vi "Decreasing temp.vi"() -> ()   [LabVIEW 2016]
uses:
  <userlib>/Levylab/LV to ITX/LVtoITX.lvclass
  <vilib>/Analysis/NI_AALPro.lvlib
panel:
  out "appended array":dbl[][](array[numeric])
  out "M vs Temp Normalized 2":cluster{dbl[], dbl[]}[](graph)
  out "M vs Temp Normalized":cluster{dbl[], dbl[]}[](graph)
  out "output cluster":cluster{dbl[], dbl[], dbl[], dbl[]}
  in  "parameter bounds 2":T1={"slope min"=-inf, "slope max"=inf, "intercept min"=-inf, "intercept max"=inf}
  out "M vs Temp":T2(graph)
  out "Fits":T2(graph)
  out "Temp vs Time":cluster{"Data":dbl[], "Data":dbl[]}(graph)
  out "G vs Temp":cluster{"Data":dbl[], "Data":dbl[]}[](graph)
  in  "Path":path
  out "Wavenames":string[](array[string])
  out "Comments":string
  in  "header length":i32=11
  out "G vs Time":cluster{"Data":dbl[], "Data":dbl[]}[](graph)
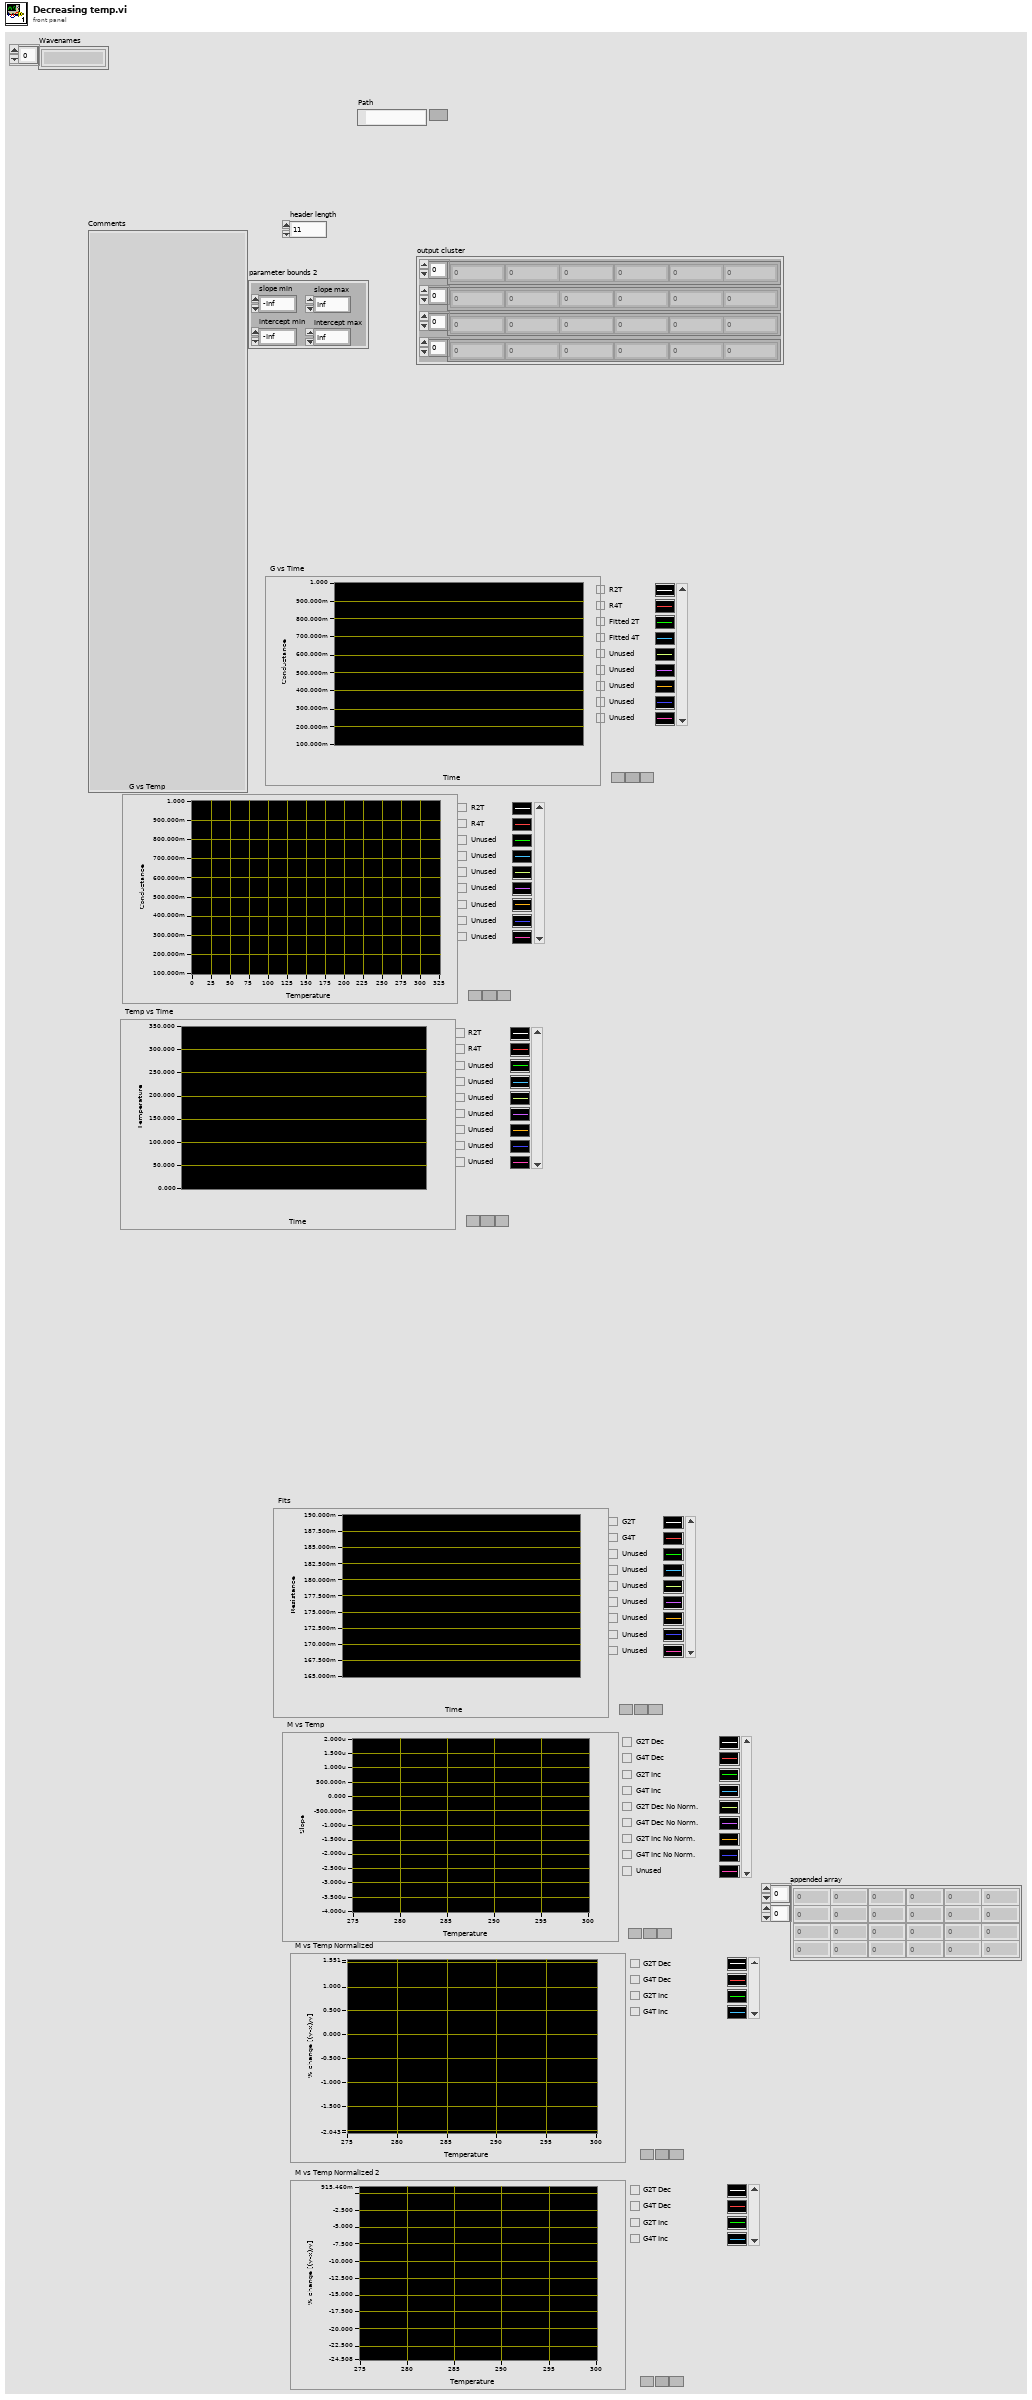
[diagram p1: front panel]
types:
  T1 = cluster{"slope min":dbl, "slope max":dbl, "intercept min":dbl, "intercept max":dbl}
  T2 = cluster{"Data":dbl[], "Best Exponential Fit":dbl[]}[]
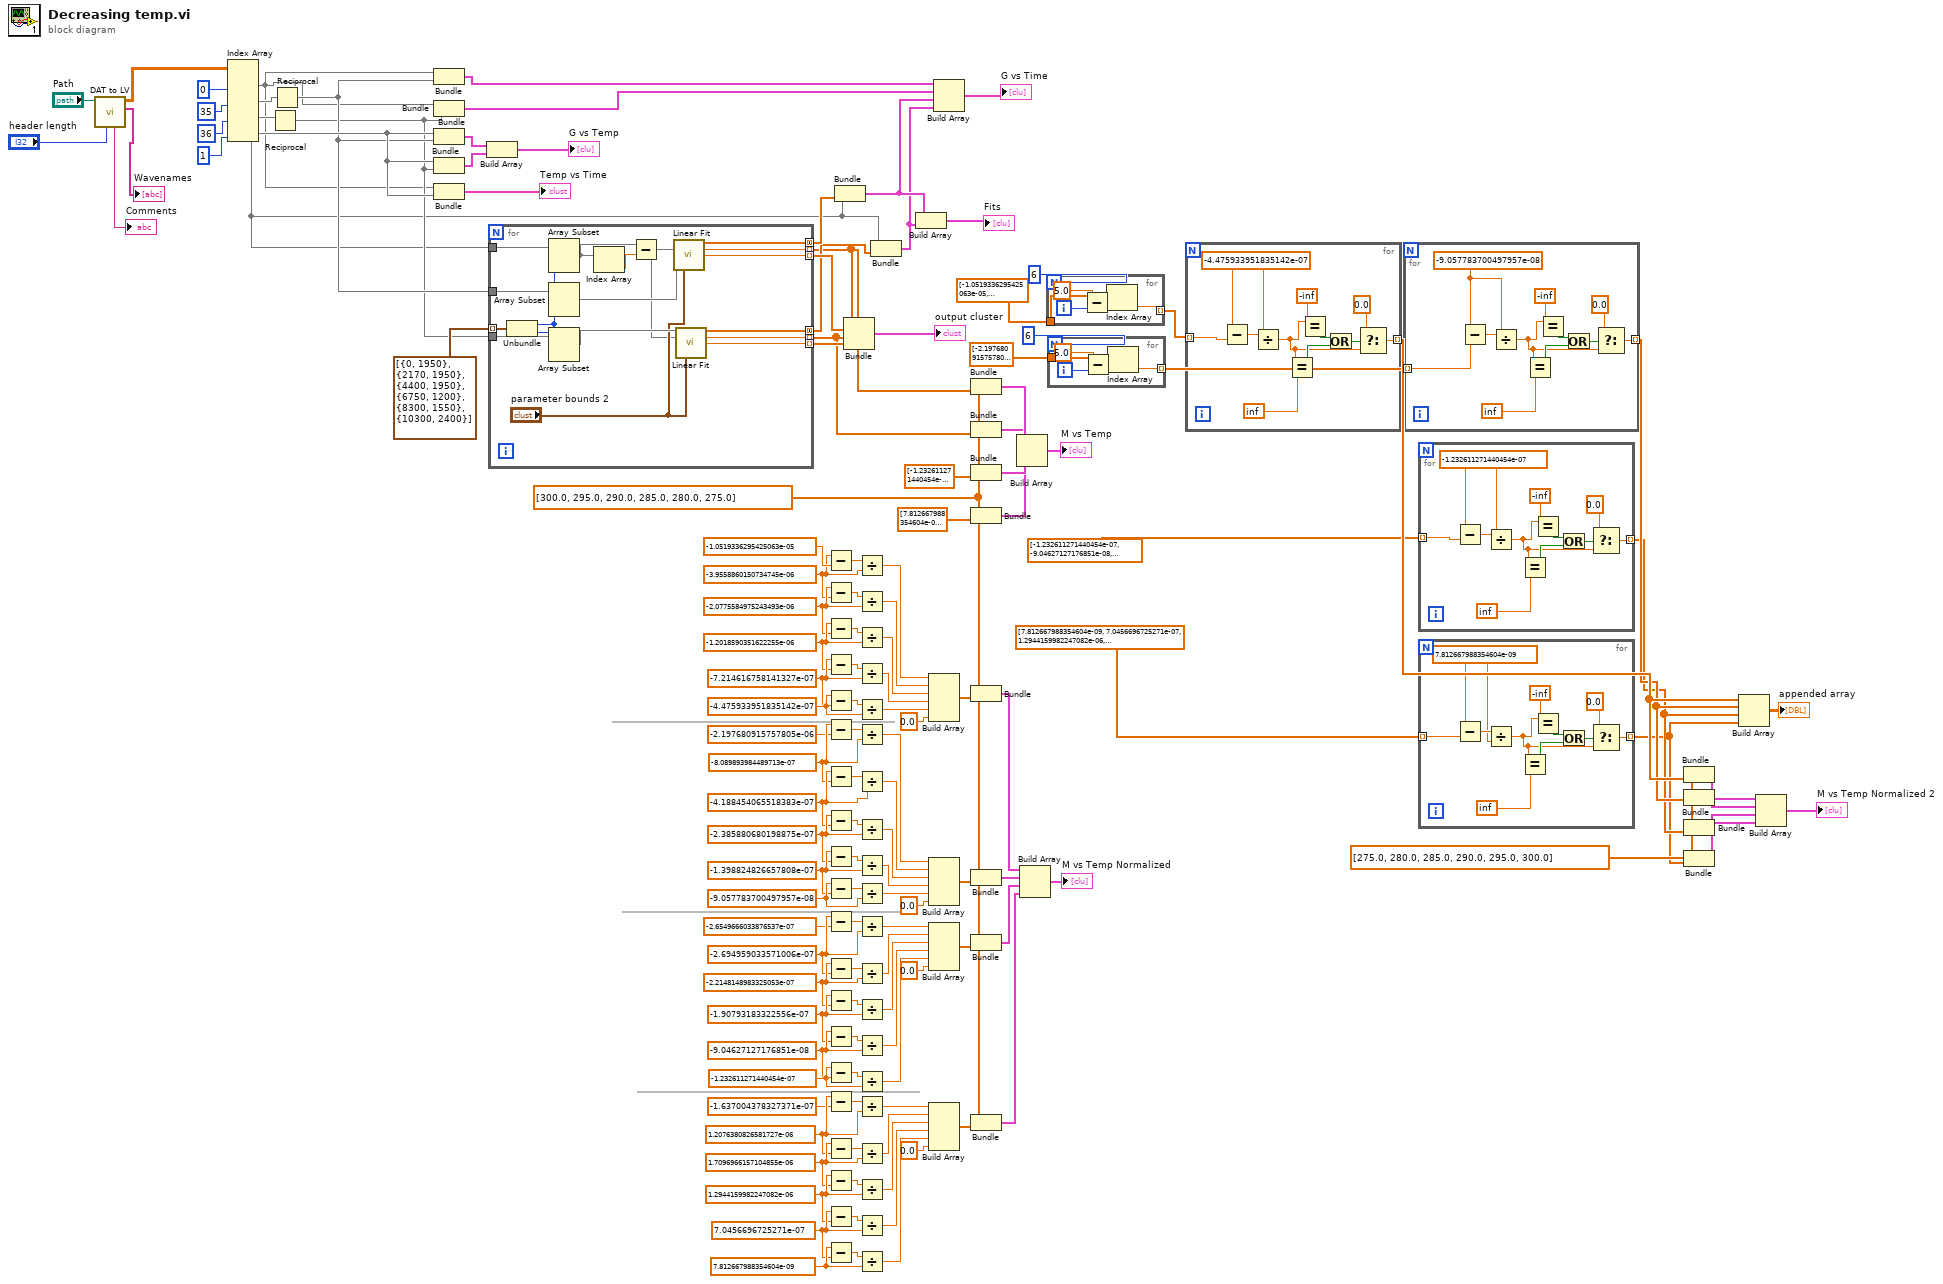
[diagram p0: block diagram]
diagram:
  w17 = dbl[] [275.0, 280.0, 285.0, 290.0, 295.0, 300.0]
  w29 = 1.2076380826581727e-06 ("slope")
  w30 = 1.7096966157104855e-06 ("slope")
  w31 = 1.2944159982247082e-06 ("slope")
  w32 = 7.0456696725271e-07 ("slope")
  w33 = 7.812667988354604e-09 ("slope")
  w46 = -2.694959033571006e-07 ("slope")
  w47 = -2.2148148983325053e-07 ("slope")
  w48 = -1.90793183322556e-07 ("slope")
  w49 = -9.04627127176851e-08 ("slope")
  w50 = -1.232611271440454e-07 ("slope")
  w67 = -9.057783700497957e-08 ("slope")
  w66 = -1.398824826657808e-07 ("slope")
  w65 = -2.385880680198875e-07 ("slope")
  w64 = -4.188454065518383e-07 ("slope")
  w63 = -8.089893984489713e-07 ("slope")
  w97 = -4.475933951835142e-07 ("slope")
  w95 = -7.214616758141327e-07 ("slope")
  w93 = -1.2018590351622255e-06 ("slope")
  w91 = -2.0775584975243493e-06 ("slope")
  w88 = -3.9558860150734745e-06 ("slope")
  w22 = dbl[] [300.0, 295.0, 290.0, 285.0, 280.0, 275.0]
  n1 = call <userlib>:"DAT to LV.vi"("header length"="header length", "File Path"="Path") -> ("Wavenames"=→"Wavenames":string[], "Data"=w129:dbl[][], "Comments"=→"Comments":string)  [unwired: 6 in, 1 out]
  n2 = Index Array(array=w129, index (col) #1=0 ("disabled index (col)"), index (col) #2=35 ("index (col)"), index (col) #3=36 ("index (col)"), index (col) #4=1 ("index (col)")) -> (element #1=w103:dbl[], element #2=w115:dbl[], element #3=w116:dbl[], element #4=w123:dbl[])  [unwired: 4 in]
  n3 = Reciprocal(x=w116) -> (1/x=w113:dbl[])
  n4 = Reciprocal(x=w115) -> (1/x=w114:dbl[])
  n5 = Bundle("Data"=w103, w114) -> (w128:cluster{"Data":dbl[], dbl[]})  [unwired: 1 in]
  n6 = Bundle("Data"=w103, w113) -> (w127:cluster{"Data":dbl[], dbl[]})  [unwired: 1 in]
  n7 = Bundle("Data"=w123, w114) -> (w125:cluster{"Data":dbl[], dbl[]})  [unwired: 1 in]
  n8 = Bundle("Data"=w123, w113) -> (w126:cluster{"Data":dbl[], dbl[]})  [unwired: 1 in]
  n9 = Bundle("Data"=w103, "Data"=w123) -> (→"Temp vs Time":cluster{"Data":dbl[], "Data":dbl[]})  [unwired: 1 in]
  n10 = Build Array(w125, w126) -> (→"G vs Temp":cluster{"Data":dbl[], dbl[]}[])
  n11 = for {
    tunnel: cluster{"index":i32, "length":i32}[] [{"index"=0, "length"=1950}, {"index"=2170, "length"=1950}, {"index"=4400, "length"=1950}, {"index"=6750, "length"=1200}, {"index"=8300, "length"=1550}, {"index"=10300, "length"=2400}] -> [w155] mode=indexing
    tunnel: [w154] -> w98 mode=indexing
    tunnel: [w153] -> w120 mode=indexing
    tunnel: [w152] -> w99 mode=indexing
    tunnel: [w151] -> w118 mode=indexing
    tunnel: [w150] -> w100 mode=concatenating
    tunnel: [w149] -> w121 mode=concatenating
    tunnel: w114 -> [w147]
    tunnel: w113 -> [w146]
    tunnel: w103 -> [w142]
    n12 = Unbundle(w155) -> ("index"=w141:i32, "length"=w148:i32)
    n13 = Array Subset(array=w142, index=w141, length=w148) -> (w139:dbl[])
    n14 = Array Subset(array=w147, index=w141, length=w148) -> (w144:dbl[])
    n15 = Array Subset(array=w146, index=w141, length=w148) -> (w145:dbl[])
    n16 = Index Array(array=w139) -> (element=w140:dbl)  [unwired: 1 in]
    n17 = Subtract(x=w139, y=w140) -> (x-y=w138:dbl[])
    n18 = call <vilib>:"Linear Fit.vi"("Y"=w144, "X"=w138, "parameter bounds"="parameter bounds 2") -> ("Best Linear Fit"=w149:dbl[], "slope"=w154:dbl, "intercept"=w153:dbl)  [unwired: 8 in, 2 out]
    n19 = call <vilib>:"Linear Fit.vi"("Y"=w145, "X"=w138, "parameter bounds"="parameter bounds 2") -> ("Best Linear Fit"=w150:dbl[], "slope"=w152:dbl, "intercept"=w151:dbl)  [unwired: 8 in, 2 out]
  }
  n20 = Subtract(x=w88, y=-1.0519336295425063e-05 ("slope")) -> (x-y=w87:dbl)
  n21 = Subtract(x=w91, y=w88) -> (x-y=w90:dbl)
  n22 = Subtract(x=w93, y=w91) -> (x-y=w92:dbl)
  n23 = Subtract(x=w95, y=w93) -> (x-y=w94:dbl)
  n24 = Subtract(x=w97, y=w95) -> (x-y=w96:dbl)
  n25 = Subtract(x=w63, y=-2.197680915757805e-06 ("slope")) -> (x-y=w72:dbl)
  n26 = Subtract(x=w64, y=w63) -> (x-y=w71:dbl)
  n27 = Subtract(x=w65, y=w64) -> (x-y=w70:dbl)
  n28 = Subtract(x=w66, y=w65) -> (x-y=w69:dbl)
  n29 = Subtract(x=w67, y=w66) -> (x-y=w68:dbl)
  n30 = Subtract(x=w46, y=-2.6549666033876537e-07 ("slope")) -> (x-y=w57:dbl)
  n31 = Subtract(x=w47, y=w46) -> (x-y=w58:dbl)
  n32 = Subtract(x=w48, y=w47) -> (x-y=w59:dbl)
  n33 = Subtract(x=w49, y=w48) -> (x-y=w60:dbl)
  n34 = Subtract(x=w50, y=w49) -> (x-y=w61:dbl)
  n35 = Subtract(x=w29, y=-1.637004378327371e-07 ("slope")) -> (x-y=w38:dbl)
  n36 = Subtract(x=w30, y=w29) -> (x-y=w37:dbl)
  n37 = Subtract(x=w31, y=w30) -> (x-y=w36:dbl)
  n38 = Subtract(x=w32, y=w31) -> (x-y=w35:dbl)
  n39 = Subtract(x=w33, y=w32) -> (x-y=w34:dbl)
  n40 = Bundle("Data"=w103, "Best Linear Fit"=w121) -> (w112:cluster{"Data":dbl[], "Best Linear Fit":dbl[]})  [unwired: 1 in]
  n41 = Bundle(w98, w120, w99, w118) -> (→"output cluster":cluster{dbl[], dbl[], dbl[], dbl[]})  [unwired: 1 in]
  n42 = Divide(x=w87, y=w88) -> (x/y=w85:dbl)
  n43 = Divide(x=w90, y=w91) -> (x/y=w84:dbl)
  n44 = Divide(x=w92, y=w93) -> (x/y=w83:dbl)
  n45 = Divide(x=w94, y=w95) -> (x/y=w82:dbl)
  n46 = Divide(x=w96, y=w97) -> (x/y=w81:dbl)
  n47 = Divide(x=w72, y=w63) -> (x/y=w74:dbl)
  n48 = Divide(x=w71, y=w64) -> (x/y=w75:dbl)
  n49 = Divide(x=w70, y=w65) -> (x/y=w76:dbl)
  n50 = Divide(x=w69, y=w66) -> (x/y=w77:dbl)
  n51 = Divide(x=w68, y=w67) -> (x/y=w78:dbl)
  n52 = Divide(x=w57, y=w46) -> (x/y=w56:dbl)
  n53 = Divide(x=w58, y=w47) -> (x/y=w55:dbl)
  n54 = Divide(x=w59, y=w48) -> (x/y=w54:dbl)
  n55 = Divide(x=w60, y=w49) -> (x/y=w53:dbl)
  n56 = Divide(x=w61, y=w50) -> (x/y=w52:dbl)
  n57 = Divide(x=w38, y=w29) -> (x/y=w39:dbl)
  n58 = Divide(x=w37, y=w30) -> (x/y=w40:dbl)
  n59 = Divide(x=w36, y=w31) -> (x/y=w41:dbl)
  n60 = Divide(x=w35, y=w32) -> (x/y=w42:dbl)
  n61 = Divide(x=w34, y=w33) -> (x/y=w43:dbl)
  n62 = Bundle("Data"=w103, "Best Linear Fit"=w100) -> (w111:cluster{"Data":dbl[], "Best Linear Fit":dbl[]})  [unwired: 1 in]
  n63 = Build Array(w112, w111) -> (→"Fits":cluster{"Data":dbl[], "Best Linear Fit":dbl[]}[])
  n64 = Build Array(w85, w84, w83, w82, w81, 0.0) -> (w86:dbl[])
  n65 = Build Array(w74, w75, w76, w77, w78, 0.0) -> (w73:dbl[])
  n66 = Build Array(w56, w55, w54, w53, w52, 0.0) -> (w25:dbl[])
  n67 = Build Array(w39, w40, w41, w42, w43, 0.0) -> (w21:dbl[])
  n68 = Build Array(w128, w127, w112, w111) -> (→"G vs Time":cluster{"Data":dbl[], "Best Linear Fit":dbl[]}[])
  n69 = Bundle(w22, w98) -> (w110:cluster{dbl[], dbl[]})  [unwired: 1 in]
  n70 = Bundle(w22, w99) -> (w105:cluster{dbl[], dbl[]})  [unwired: 1 in]
  n71 = Bundle(w22, "2T Slope"=dbl[] [-1.232611271440454e-07, -9.04627127176851e-08, -1.90793183322556e-07, -2.2148148983325053e-07, -2.694959033571006e-07, -2.6549666033876537e-07]) -> (w109:cluster{dbl[], "2T Slope":dbl[]})  [unwired: 1 in]
  n72 = Bundle(w22, "4T Slope"=dbl[] [7.812667988354604e-09, 7.0456696725271e-07, 1.2944159982247082e-06, 1.7096966157104855e-06, 1.2076380826581727e-06, -1.637004378327371e-07]) -> (w108:cluster{dbl[], "4T Slope":dbl[]})  [unwired: 1 in]
  n73 = Bundle(w22, w86) -> (w27:cluster{dbl[], dbl[]})  [unwired: 1 in]
  n74 = Bundle(w22, w73) -> (w26:cluster{dbl[], dbl[]})  [unwired: 1 in]
  n75 = Bundle(w22, w25) -> (w24:cluster{dbl[], dbl[]})  [unwired: 1 in]
  n76 = Bundle(w22, w21) -> (w23:cluster{dbl[], dbl[]})  [unwired: 1 in]
  n77 = Build Array(w110, w105, w109, w108) -> (→"M vs Temp":cluster{dbl[], "4T Slope":dbl[]}[])
  n78 = Build Array(w27, w26, w24, w23) -> (→"M vs Temp Normalized":cluster{dbl[], dbl[]}[])
  n79 = for {
    N: 6 -> [_]
    tunnel: [w160] -> w2 mode=indexing
    tunnel: dbl[] [-1.0519336295425063e-05, -3.9558860150734745e-06, -2.0775584975243493e-06, -1.2018590351622255e-06, -7.214616758141327e-07, -4.475933951835142e-07] ("Array") -> [w156]
    i -> [w158]
    n80 = Subtract(x=5.0, y=w158) -> (x-y=w157:dbl)
    n81 = Index Array(array=w156, index=w157) -> (element=w160:dbl)
  }
  n82 = for {
    N: 6 -> [_]
    tunnel: dbl[] [-2.197680915757805e-06, -8.089893984489713e-07, -4.188454065518383e-07, -2.385880680198875e-07, -1.398824826657808e-07, -9.057783700497957e-08] ("Array 2") -> [w165]
    tunnel: [w161] -> w1 mode=indexing
    i -> [w163]
    n83 = Subtract(x=5.0, y=w163) -> (x-y=w162:dbl)
    n84 = Index Array(array=w165, index=w162) -> (element=w161:dbl)
  }
  n85 = for {
    tunnel: w2 -> [w175] mode=indexing
    tunnel: [w173] -> w11 mode=indexing
    w166 = -4.475933951835142e-07 ("slope")
    n86 = Subtract(x=w166, y=w175) -> (x-y=w176:dbl)
    n87 = Divide(x=w176, y=w166) -> (x/y=w168:dbl)
    n88 = Equal?(x=w168, y=inf) -> (x = y?=w170:bool)
    n89 = Equal?(x=w168, y=-inf) -> (x = y?=w169:bool)
    n90 = Or(x=w169, y=w170) -> (x .or. y?=w167:bool)
    n91 = Select(t=0.0, s=w167, f=w168) -> (s? t:f=w173:dbl)
  }
  n92 = for {
    tunnel: [w185] -> w10 mode=indexing
    tunnel: w1 -> [w177] mode=indexing
    w178 = -9.057783700497957e-08 ("slope")
    n93 = Subtract(x=w178, y=w177) -> (x-y=w187:dbl)
    n94 = Divide(x=w187, y=w178) -> (x/y=w180:dbl)
    n95 = Equal?(x=w180, y=inf) -> (x = y?=w182:bool)
    n96 = Equal?(x=w180, y=-inf) -> (x = y?=w181:bool)
    n97 = Or(x=w181, y=w182) -> (x .or. y?=w179:bool)
    n98 = Select(t=0.0, s=w179, f=w180) -> (s? t:f=w185:dbl)
  }
  n99 = for {
    tunnel: dbl[] [-1.232611271440454e-07, -9.04627127176851e-08, -1.90793183322556e-07, -2.2148148983325053e-07, -2.694959033571006e-07, -2.6549666033876537e-07] ("2T Slope") -> [w197] mode=indexing
    tunnel: [w195] -> w9 mode=indexing
    w188 = -1.232611271440454e-07 ("slope")
    n100 = Subtract(x=w188, y=w197) -> (x-y=w198:dbl)
    n101 = Divide(x=w198, y=w188) -> (x/y=w190:dbl)
    n102 = Equal?(x=w190, y=inf) -> (x = y?=w192:bool)
    n103 = Equal?(x=w190, y=-inf) -> (x = y?=w191:bool)
    n104 = Or(x=w191, y=w192) -> (x .or. y?=w189:bool)
    n105 = Select(t=0.0, s=w189, f=w190) -> (s? t:f=w195:dbl)
  }
  n106 = for {
    tunnel: [w207] -> w8 mode=indexing
    tunnel: dbl[] [7.812667988354604e-09, 7.0456696725271e-07, 1.2944159982247082e-06, 1.7096966157104855e-06, 1.2076380826581727e-06, -1.637004378327371e-07] ("4T Slope") -> [w200] mode=indexing
    w199 = 7.812667988354604e-09 ("slope")
    n107 = Subtract(x=w199, y=w200) -> (x-y=w209:dbl)
    n108 = Divide(x=w209, y=w199) -> (x/y=w202:dbl)
    n109 = Equal?(x=w202, y=inf) -> (x = y?=w204:bool)
    n110 = Equal?(x=w202, y=-inf) -> (x = y?=w203:bool)
    n111 = Or(x=w203, y=w204) -> (x .or. y?=w201:bool)
    n112 = Select(t=0.0, s=w201, f=w202) -> (s? t:f=w207:dbl)
  }
  n113 = Bundle(w17, w11) -> (w16:cluster{dbl[], dbl[]})  [unwired: 1 in]
  n114 = Bundle(w17, w10) -> (w15:cluster{dbl[], dbl[]})  [unwired: 1 in]
  n115 = Bundle(w17, w9) -> (w14:cluster{dbl[], dbl[]})  [unwired: 1 in]
  n116 = Bundle(w17, w8) -> (w13:cluster{dbl[], dbl[]})  [unwired: 1 in]
  n117 = Build Array(w11, w10, w9, w8) -> (→"appended array":dbl[][])
  n118 = Build Array(w16, w15, w14, w13) -> (→"M vs Temp Normalized 2":cluster{dbl[], dbl[]}[])
